vi "Traverse-Settings-Save.vi"() -> ()   [LabVIEW 2017]
uses:
  Settings-Control.ctl
panel:
  in  "Settings":T1
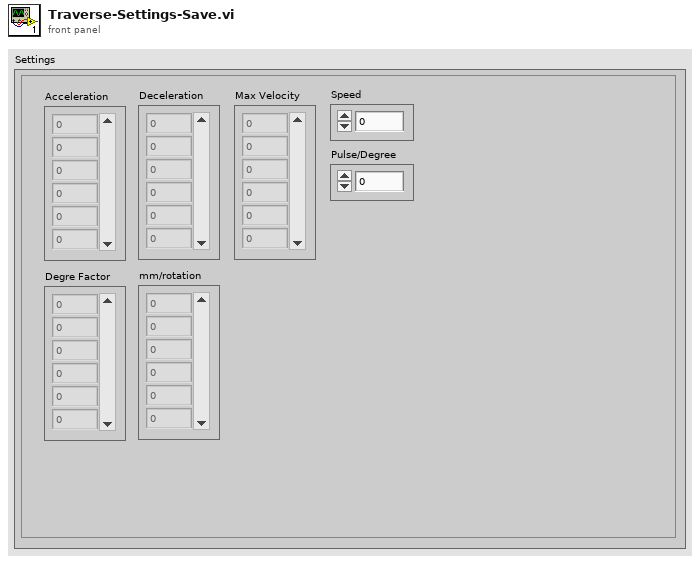
[diagram p1: front panel]
types:
  T1 = typedef "Settings-Control.ctl" = cluster{"Acceleration":dbl[], "Deceleration":dbl[], "Max Velocity":dbl[], "Speed":dbl, "Pulse/Degree":dbl, "Degre Factor":dbl[], "mm/rotation":dbl[]}
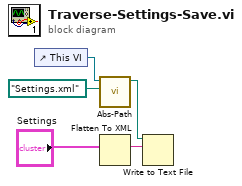
[diagram p0: block diagram]
diagram:
  n1 = control-ref of="This VI"() -> (w4:refnum<vi>)
  n2 = call "Abs-Path.vi"("filename"=path "Settings.xml" ("file (use dialog)"), "Vi in path"=w4) -> ("Full path"=w2:path)  [unwired: 9 in]
  n3 = Flatten To XML(anything="Settings") -> (xml string=w5:string)
  n4 = Write to Text File(file (use dialog)=w2, text=w5) -> ()  [unwired: 2 in, 3 out]
